vi "PMA Manuell Kalibrieren.vi"(8 "GT":bool, 10 "Kalibrieren":T4, 11 "AUTO STARTEN":bool) -> (2 "Wert im gültigen Bereich:":bool, 3 "Kalibrieren erfolgreich":bool)   [LabVIEW 2020, in "ABB-EL3000.lvlib" / "PMA.lvlib" / "Kalibrieren.lvlib"]
uses:
  Kalibrieren.lvlib
  Visualisierungs Elemente/Button.ctl
  Kalibrierung O2.ctl
  Visualisierungs Elemente/String - Ausgabefeld.ctl
  Visualisierungs Elemente/Zahlen-Ausgabefeld.ctl
  Analysator Definition/FGV Analysator Definition Aktionen.ctl
  Sprachverwaltung/FGV Aktion Tabelle zerlegen.ctl
  CalGas Aufschaltung/FGV CalGas Aktionen.ctl
  Linearisierung V2/Aktion Lin Daten aufarbeiten.ctl
  Allgemeine VI/FGV Uras26 Aktion.ctl
  Allgemeine VI/Allgemeine VI.lvlib
  Auto Kalibrieren/Auto Kalibrieren.lvlib
  Analysator Definition/Analysator Definition.lvlib
  CalGas Aufschaltung/CalGas Aufschaltung.lvlib
  Sprachverwaltung/Sprachverwaltung.lvlib
  Allgemein/allgemeine Sub-VIs.lvlib
  Linearisierung V2/Linearisierung v2.lvlib
panel:
  in  "Speichern":T1
  in  "Kalibrierwerte kopieren?:":bool
  out "Titelzeile":string
  out "Roh Wert O2:":T2 format="%.3f"
  out "Status":T3
  in  "Konzentration":sgl format="%#_5g"
  out "Messbereich":T3
  in  "STARTEN":bool
  in  "ABBRECHEN":T1
  # "Messbereich"
  # "%"
  # "Konzentration"
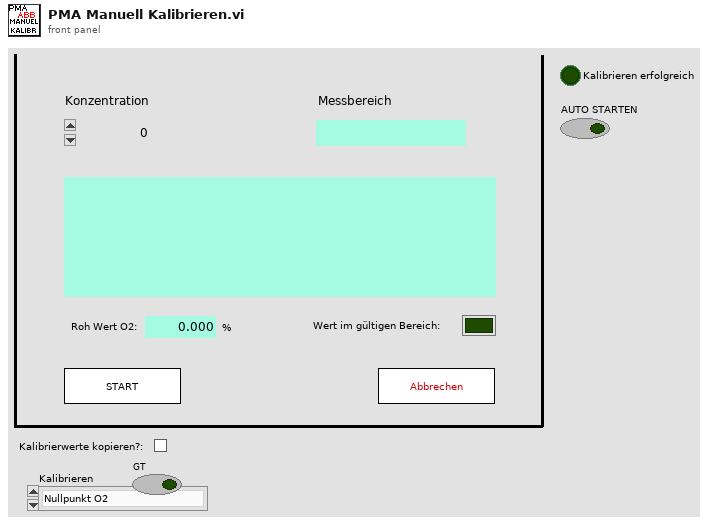
[diagram p1: front panel]
types:
  T1 = typedef "Button.ctl" = bool
  T2 = typedef "Zahlen-Ausgabefeld.ctl" = sgl
  T3 = typedef "String - Ausgabefeld.ctl" = string
  T4 = typedef "ABB-EL3000.lvlib/PMA.lvlib/Kalibrieren.lvlib/Kalibrierung O2.ctl" = enum16{"Nullpunkt O2", "Endpunkt O2"}
  T5 = typedef "Sprachverwaltung.lvlib/FGV Aktion Tabelle zerlegen.ctl" = enum16{"laden", "vereinzeln", "speichern"}
  T6 = enum8{"Enabled", "Disabled", "Disabled and Grayed Out"}
  T7 = typedef "Analysator Definition.lvlib/FGV Analysator Definition Aktionen.ctl" = enum16{"lesen", "MB setzen", "MB KAL setzen", "laden"}
  T8 = typedef "Linearisierung v2.lvlib/Aktion Lin Daten aufarbeiten.ctl" = enum16{"lesen", "Protkolldaten", "speichern", "laden", "EPA auswerten", "Tabelle schreiben", "Lin auswerten", "Tab init", "Stufentabelle", "EPA aktiviert", "Nachbehandlung laden", "Tabelle löschen", "Istwerte löschen", "Zeile löschen", "Zeile einfügen", "LIN aktiviert", "LIN/EPA aktiv laden", "EGAK Tab", "LIN übernehmen", "Tab init ohne Stufen"}
  T9 = typedef "CalGas Aufschaltung.lvlib/FGV CalGas Aktionen.ctl" = enum16{"lesen", "Analysator Auswahl", "Def.CalGas", "Aufschaltung CalGas", "laden", "speichern", "KAL extrahieren"}
  T10 = typedef "Linearisierung v2.lvlib/Lin-Polynom Daten.ctl" = cluster{"Messgerät":string, "Kalibrator (Gasteiler)":string, "Bearbeiter/in":string, "Komponente":string, "Zeitstempel":timestamp, "F_max gefordert (%)":sgl, "F_max in %":sgl, "F_max in ppm":sgl, "Vorschlag Ordnung":i32, "Polynom OK":bool, "Polynomkoeff.":dbl[], "Prüfgas Konzentration":dbl, "Pfad EPA":string, "Pfad_LIN":string, "Gasnummer:":u8, "Komponentenauswahl":T11, "Verdünnungsgas":T13, "Zeitdauer Stufe":T14, "Anzahl Stufen":T14, "F_max in % EPA":sgl, "F_max in ppm EPA":sgl, "F_max in % LIN":sgl, "F_max in ppm LIN":sgl, "Punkte umkehren":bool, "EPA Optionsfeld":T15, "Autolin Hovacal":T16, "Spanfactors":sgl[], "Kalibrierauswahl":T17, "Conditions:":T18, "Gasflaschen Nr.:":string, "Bottle Accuracy":dbl, "Konfig Gasflasche":T19, "Gasflasche":T20, "HovaCAL Flow AutoLin":T21, "MFC Output":T22, "Gas Ablaufdatum":timestamp, "Lin Modus":T23, "zusätzliche Zeitdauer Erster Punkt":sgl, "Offsets":sgl[]}
  T11 = typedef "Linearisierung v2.lvlib/KomponentenArray.ctl" = cluster{"Komponente:":T12, "Konzentration":dbl}[]
  T12 = typedef "Auswahlfeld.ctl" = u16
  T13 = typedef "Linearisierung v2.lvlib/Gasteiler.lvlib/Prüfgas in.ctl" = u16
  T14 = typedef "Zahlen-Eingabefeld.ctl" = sgl
  T15 = typedef "Linearisierung v2.lvlib/EPA Optionsfeld.ctl" = enum32{"Istwert", "Rohwert", "Linearisierter Wert"}
  T16 = typedef "Linearisierung v2.lvlib/Gasteiler.lvlib/HovaCal.lvlib/AutoLin Hovacal.ctl" = enum32{"Keine Auswahl", "Optionsauswahl 1", "Optionsauswahl 2"}
  T17 = typedef "Linearisierung v2.lvlib/Kalibrieroption.ctl" = u16
  T18 = typedef "Linearisierung v2.lvlib/Linearity verification 1065-307.lvlib/Condition.ctl" = u16
  T19 = typedef "System Einstellungen V2.lvlib/Konfig Gasflasche.ctl" = bool
  T20 = typedef "System Einstellungen V2.lvlib/Gasflasche Auswahl.ctl" = u16
  T21 = typedef "Linearisierung v2.lvlib/Gasteiler.lvlib/HovaCAL_Interface.lvlib/Controls.lvlib/Flow Einstellung.ctl" = cluster{"HovaCAL Flow Input Cluster":dbl}
  T22 = typedef "Linearisierung v2.lvlib/Gasteiler.lvlib/HovaCAL_Interface.lvlib/Controls.lvlib/Pump state.ctl" = cluster{"Run":bool}
  T23 = typedef "CalGas Aufschaltung.lvlib/Lin Modus.ctl" = u16
  T24 = typedef "CalGas Aufschaltung.lvlib/Definition CalGas Anzeige.ctl" = cluster{"Namen":T25, "Werte":T27, "Werte 2":T27, "Einheit":T28, "Messbereiche":T29}
  T25 = typedef "CalGas Aufschaltung.lvlib/CalGas-Namen.ctl" = cluster{"Name":T26, "Name 2":T26, "Name 3":T26, "Name 4":T26, "Name 5":T26, "Name 6":T26, "Name 7":T26, "Name 8":T26, "Name 9":T26, "Name 10":T26, "Name 11":T26, "Name 12":T26}
  T26 = typedef "String - Eingabefeld.ctl" = string
  T27 = typedef "CalGas Aufschaltung.lvlib/CalGas-Werte.ctl" = cluster{"Konzentration 1":T14, "Konzentration 2":T14, "Konzentration 3":T14, "Konzentration 4":T14, "Konzentration 5":T14, "Konzentration 6":T14, "Konzentration 7":T14, "Konzentration 8":T14, "Konzentration 9":T14, "Konzentration 10":T14, "Konzentration 11":T14, "Konzentration 12":T14}
  T28 = typedef "CalGas Aufschaltung.lvlib/CalGas-Einheit.ctl" = cluster{"Einheit 1":T12, "Einheit 2":T12, "Einheit 3":T12, "Einheit 4":T12, "Einheit 5":T12, "Einheit 6":T12, "Einheit 7":T12, "Einheit 8":T12, "Einheit 9":T12, "Einheit 10":T12, "Einheit 11":T12, "Einheit 12":T12}
  T29 = typedef "CalGas Aufschaltung.lvlib/CalGas-Messbereiche.ctl" = cluster{"Messbereich 1":T12, "Messbereich 2":T12, "Messbereich 3":T12, "Messbereich 4":T12, "Messbereich 5":T12, "Messbereich 6":T12, "Messbereich 7":T12, "Messbereich 8":T12, "Messbereich 9":T12, "Messbereich 10":T12, "Messbereich 11":T12, "Messbereich 12":T12}
  T30 = typedef "Analysator Definition.lvlib/Betriebsdaten Komponente.ctl" = cluster{"Namen":string[], "MB Namen":string[], "Einheit":string, "MB Aktuell":u16, "MB Endwert":u16, "CalGase":u16[], "MB für KAL":u16[], "CG für KAL":u16[]}
  T31 = typedef "ABB-EL3000.lvlib/Allgemeine VI.lvlib/FGV Uras26 Aktion.ctl" = enum16{"lesen", "CAL-Daten laden", "Messen", "Kalibrieren vorbereiten", "Kalibrieren", "CAL-Daten speichern", "Toleranz schreiben", "CAL-Daten kopieren"}
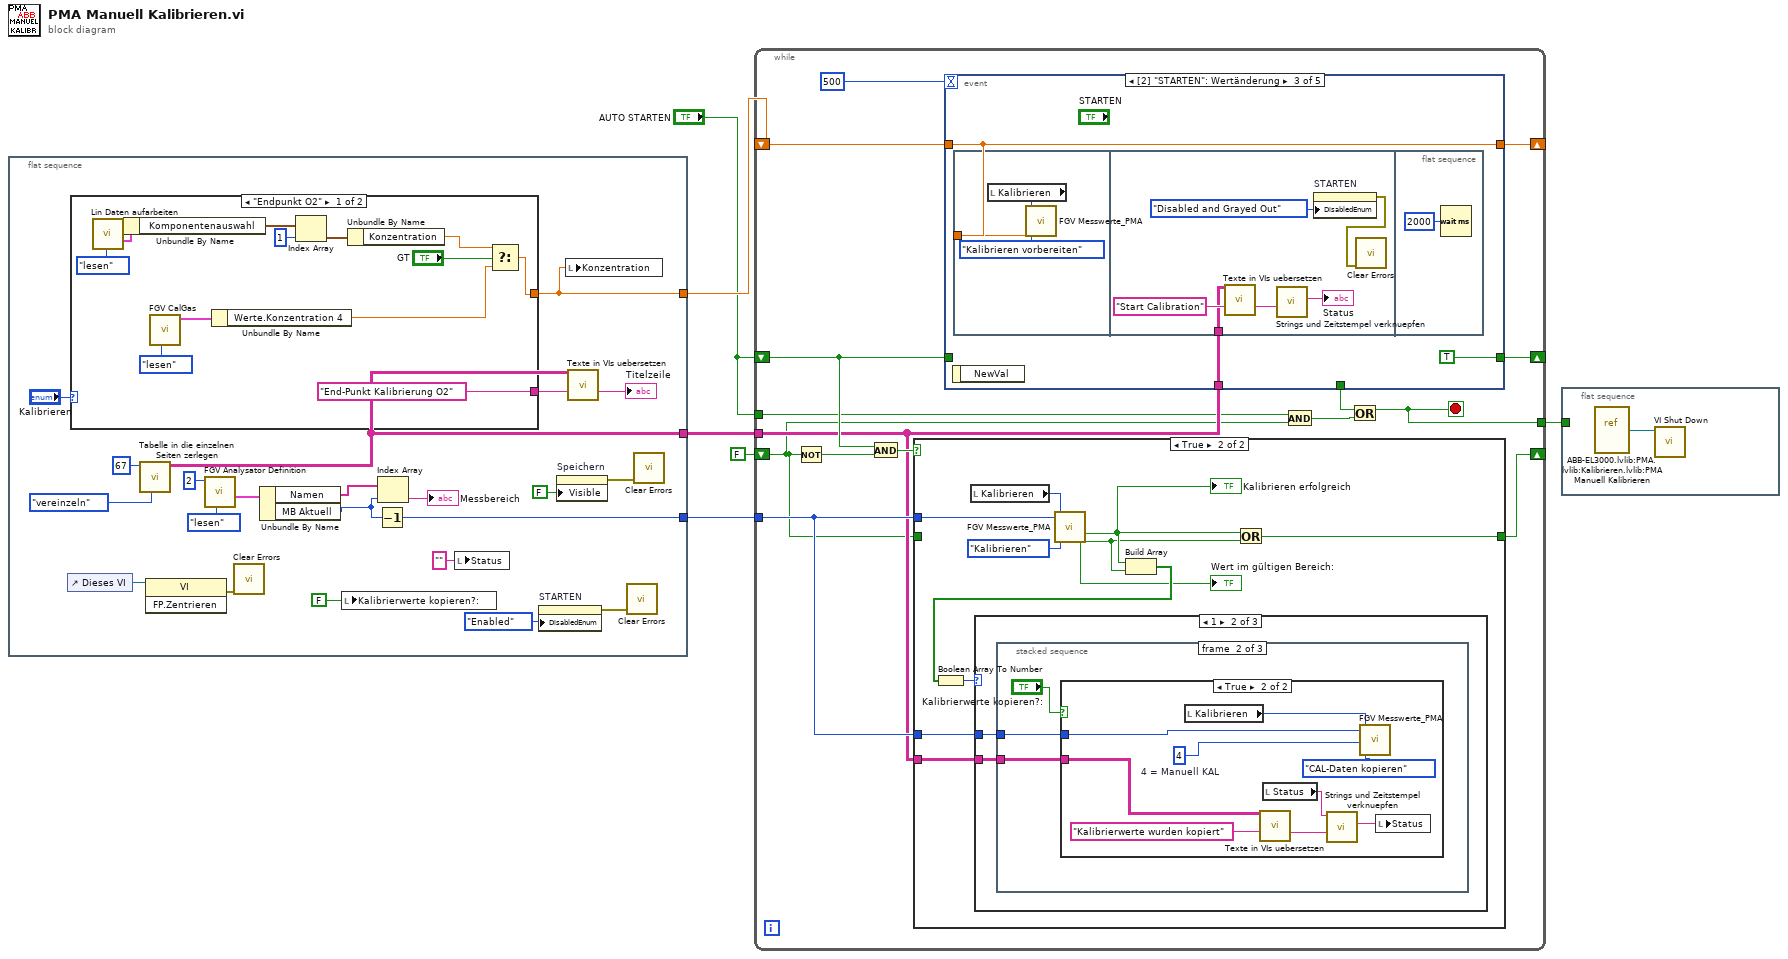
[diagram p0: block diagram]
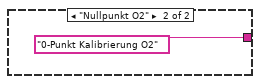
[diagram p2: hidden frame]
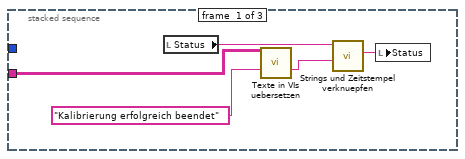
[diagram p5: hidden frame]
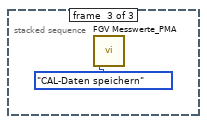
[diagram p7: hidden frame]
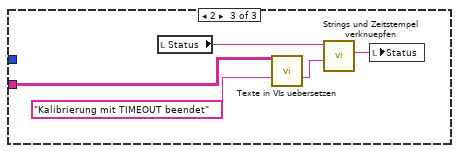
[diagram p8: hidden frame]
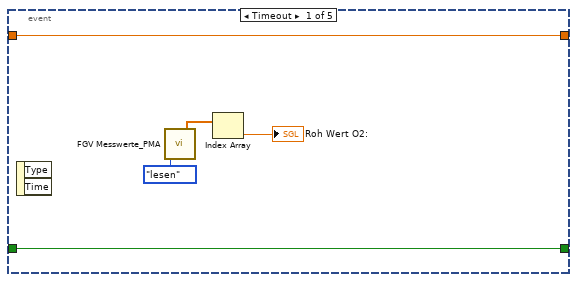
[diagram p9: hidden frame]
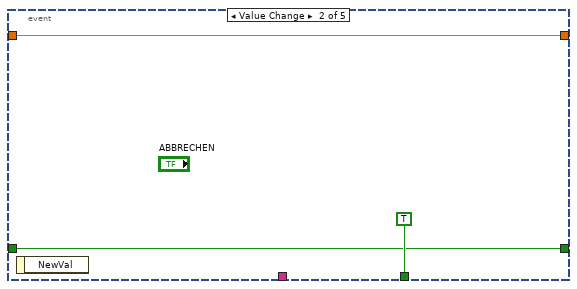
[diagram p10: hidden frame]
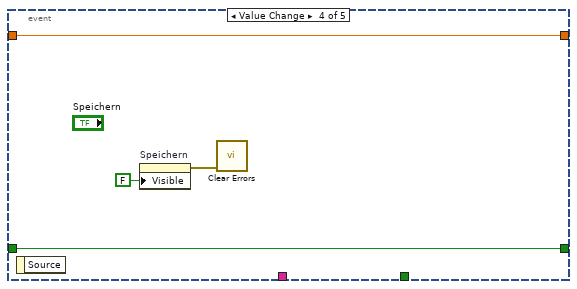
[diagram p11: hidden frame]
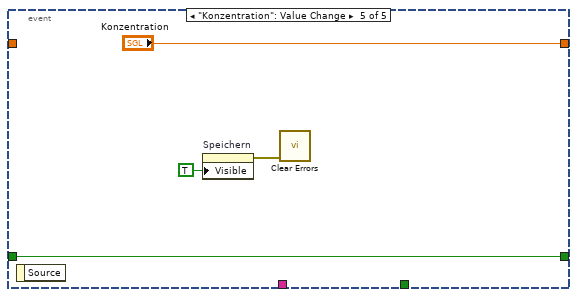
[diagram p12: hidden frame]
diagram:
  n1 = flat-sequence {
    tunnel: [w15] -> w5
    tunnel: [w8] -> w4
    tunnel: [w9] -> w3
    frame #0 {
      n2 = control-ref of="Dieses VI"() -> (w14:refnum<vi>)
      n3 = case shown="\"Endpunkt O2\"" "Kalibrieren" {
        tunnel: ["End-Punkt Kalibrierung O2" "0-Punkt Kalibrierung O2"] -> w11
        tunnel: [w29 _] -> w8
        frame "Endpunkt O2" {
          n4 = call "Lin Daten aufarbeiten.vi"("Aktionen"=Aktion_Lin_Daten_aufarbeiten."lesen") -> ("Lin-Polynom"=w32:T10)  [unwired: 16 in, 10 out]
          n5 = Unbundle By Name(w32) -> ("Komponentenauswahl"=w33:T11)
          n6 = call "FGV CalGas.vi"("Aktionen"=FGV_CalGas_Aktionen."lesen") -> ("Def.CalGas"=w38:T24)  [unwired: 6 in, 4 out]
          n7 = Unbundle By Name(w38) -> ("Werte.Konzentration 4"=w30:T14)
          n8 = Index Array(array=w33, index=1 ("Index")) -> (element=w35:cluster{"Komponente:":T12, "Konzentration":dbl})
          n9 = Unbundle By Name(w35) -> ("Konzentration"=w36:dbl)
          n10 = Select(t=w36, s="GT", f=w30) -> (s? t:f=w29:dbl)
        }
        frame "Nullpunkt O2" {
        }
      }
      n11 = call "Tabelle in die einzelnen Seiten zerlegen.vi"("Aktion"=FGV_Aktion_Tabelle_zerlegen."vereinzeln", "Index (Seite)"=67) -> ("Sprachliste"=w9:string[][])  [unwired: 7 in, 2 out]
      n12 = invoke class="VI" method="FP.Zentrieren"(reference=w14) -> (error out=w13:errorcluster)  [unwired: 2 in, 2 out]
      n13 = call "FGV Analysator Definition.vi"("Aktionen"=FGV_Analysator_Definition_Aktionen."lesen", "Komponente"=2) -> ("Betriebsdaten Komponente"=w24:T30)  [unwired: 5 in, 4 out]
      n14 = call <vilib>:"Clear Errors.vi"("error in (no error)"=w13) -> ()  [unwired: 5 in, 2 out]
      n15 = Unbundle By Name(w24) -> ("Namen"=w25:string[], "MB Aktuell"=w20:u16)
      n16 = local write "Kalibrierwerte kopieren?:"(FALSE) -> ()
      n17 = Decrement(x=w20) -> (x-1=w15:u16)
      n18 = Index Array(array=w25, index=w20) -> (element=→"Messbereich":string)
      n19 = local write "Status"(T3 "" ("Status")) -> ()
      n20 = property on="STARTEN" class="Bool."("DisabledEnum"=T6."Enabled" ("Deaktiviert")) -> (error out=w16:errorcluster)  [unwired: 2 in, 1 out]
      n21 = property on="Speichern" class="Bool."("Visible"=FALSE ("Sichtbar")) -> (error out=w19:errorcluster)  [unwired: 2 in, 1 out]
      n22 = local write "Konzentration"(w8) -> ()
      n23 = call "Texte in VIs uebersetzen.vi"("Sprachliste"=w9, "String zum Übersetzen"=w11) -> ("String zum Übersetzen"=→"Titelzeile":string)  [unwired: 9 in, 4 out]
      n24 = call <vilib>:"Clear Errors.vi"("error in (no error)"=w16) -> ()  [unwired: 5 in, 2 out]
      n25 = call <vilib>:"Clear Errors.vi"("error in (no error)"=w19) -> ()  [unwired: 5 in, 2 out]
    }
  }
  n26 = while {
    shift-right: [w55] -> _
    shift-left: "AUTO STARTEN" -> [w53]
    tunnel: w5 -> [w50]
    shift-right: [w43] -> _
    shift-left: FALSE -> [w42]
    tunnel: [w46] -> w6
    shift-right: [w49] -> _
    shift-left: w4 -> [w48]
    tunnel: w3 -> [w47]
    tunnel: "AUTO STARTEN" -> [w44]
    stop <- w46 stop-if-true
    n27 = Not(x=w42) -> (.not. x?=w54:bool)
    n28 = And(x=w53, y=w54) -> (x .and. y?=w52:bool)
    n29 = case shown="True" w52 {
      tunnel: w50 -> [_ w61]
      tunnel: [w57 w67] -> w43
      tunnel: w42 -> [w57 _]
      tunnel: w50 -> [_ w60]
      tunnel: w47 -> [_ w58]
      frame False {
      }
      frame True {
        n30 = local read "Kalibrieren"() -> (w62:T4)
        n31 = call "FGV Messwerte_PMA.vi"("Messbereich"=w61, "Kalibrieren"=w62, "Aktion"=FGV_Uras26_Aktion."Kalibrieren") -> ("im gültigen Bereich"=→"Wert im gültigen Bereich:":bool, "Kalibrieren erfolgreich"=w66:bool, "CAL TimeOut"=w65:bool)  [unwired: 17 in, 5 out]
        "Kalibrieren erfolgreich" <- w66
        n32 = Build Array(w66, w65) -> (w64:bool[])
        n33 = Boolean Array To Number(Boolean array=w64) -> (number=w63:u32)
        n34 = case shown="1" w63 {
          tunnel: w60 -> [_ w70 _]
          tunnel: w58 -> [_ w69 w89]
          frame 0, Default {
          }
          frame 1 {
            n35 = stacked-sequence {
              tunnel: w70 -> [_ w77 _]
              tunnel: w69 -> [w71 w76 _]
              frame #0 {
                n36 = local read "Status"() -> (w74:T3)
                n37 = call "Texte in VIs uebersetzen.vi"("Sprachliste"=w71, "String zum Übersetzen"="Kalibrierung erfolgreich beendet" ("String 1 hinzufügen")) -> ("String zum Übersetzen"=w72:string)  [unwired: 9 in, 4 out]
                n38 = call "Strings und Zeitstempel verknuepfen.vi"("String 1 hinzufügen"=w72, "Eingagns String"=w74) -> ("Verknüpfter String"=w75:string)  [unwired: 9 in]
                n39 = local write "Status"(w75) -> ()
              }
              frame #1 {
                n40 = case shown="True" "Kalibrierwerte kopieren?:" {
                  tunnel: w77 -> [_ w83]
                  tunnel: w76 -> [_ w79]
                  frame False {
                  }
                  frame True {
                    w82 = u16 4  # 4 = Manuell KAL
                    n41 = local read "Kalibrieren"() -> (w84:T4)
                    n42 = call "Texte in VIs uebersetzen.vi"("Sprachliste"=w79, "String zum Übersetzen"="Kalibrierwerte wurden kopiert" ("String 1 hinzufügen")) -> ("String zum Übersetzen"=w80:string)  [unwired: 9 in, 4 out]
                    n43 = local read "Status"() -> (w86:T3)
                    n44 = call "Strings und Zeitstempel verknuepfen.vi"("String 1 hinzufügen"=w80, "Eingagns String"=w86) -> ("Verknüpfter String"=w87:string)  [unwired: 9 in]
                    n45 = call "FGV Messwerte_PMA.vi"("Messbereich"=w83, "Zielmessbereich"=w82, "Kalibrieren"=w84, "Aktion"=FGV_Uras26_Aktion."CAL-Daten kopieren") -> ()  [unwired: 16 in, 8 out]
                    n46 = local write "Status"(w87) -> ()
                  }
                }
              }
              frame #2 {
                n47 = call "FGV Messwerte_PMA.vi"("Aktion"=FGV_Uras26_Aktion."CAL-Daten speichern") -> ()  [unwired: 19 in, 8 out]
              }
            }
          }
          frame 2 {
            n48 = local read "Status"() -> (w93:T3)
            n49 = call "Texte in VIs uebersetzen.vi"("Sprachliste"=w89, "String zum Übersetzen"="Kalibrierung mit TIMEOUT beendet" ("String 1 hinzufügen")) -> ("String zum Übersetzen"=w90:string)  [unwired: 9 in, 4 out]
            n50 = call "Strings und Zeitstempel verknuepfen.vi"("String 1 hinzufügen"=w90, "Eingagns String"=w93) -> ("Verknüpfter String"=w92:string)  [unwired: 9 in]
            n51 = local write "Status"(w92) -> ()
          }
        }
        n52 = Or(x=w66, y=w65) -> (x .or. y?=w67:bool)
      }
    }
    n53 = event shown="[2] \"STARTEN\": Wertänderung" {
      selector: _ -> [_ _ _ _ _]
      dyn-events: _ -> [_ _ _ _ _]
      timeout: 500 -> [_ _ _ _ _]
      tunnel: [_ TRUE ("ABBRECHEN") _ _ _] -> w51
      tunnel: [w98 w100 TRUE ("STARTEN") w117 w119] -> w55
      tunnel: w53 -> [w98 w100 _ w117 w119]
      tunnel: [w95 w99 w103 w118 "Konzentration"] -> w49
      tunnel: w48 -> [w95 w99 w103 w118 _]
      tunnel: w47 -> [_ _ w102 _ _]
      event Timeout {
        n54 = event-data() -> ()  [unwired: 1 in, 2 out]
        n55 = call "FGV Messwerte_PMA.vi"("Aktion"=FGV_Uras26_Aktion."lesen") -> ("Rohwerte"=w96:sgl[])  [unwired: 19 in, 7 out]
        n56 = Index Array(array=w96) -> (element=→"Roh Wert O2:":sgl)  [unwired: 1 in]
      }
      event Value Change {
        n57 = event-data() -> ()  [unwired: 1 in, 1 out]
      }
      event "STARTEN": Value Change {
        n58 = event-data() -> ()  [unwired: 1 in, 1 out]
        n59 = flat-sequence {
          tunnel: w103 -> [w105]
          tunnel: w102 -> [w108]
          frame #0 {
            n60 = local read "Kalibrieren"() -> (w106:T4)
            n61 = call "FGV Messwerte_PMA.vi"("Prüfgaskonz."=w105, "Kalibrieren"=w106, "Aktion"=FGV_Uras26_Aktion."Kalibrieren vorbereiten") -> ()  [unwired: 17 in, 8 out]
          }
          frame #1 {
            n62 = call "Texte in VIs uebersetzen.vi"("Sprachliste"=w108, "String zum Übersetzen"="Start Calibration" ("String 1 hinzufügen")) -> ("String zum Übersetzen"=w109:string)  [unwired: 9 in, 4 out]
            n63 = call "Strings und Zeitstempel verknuepfen.vi"("String 1 hinzufügen"=w109) -> ("Verknüpfter String"=→"Status":string)  [unwired: 10 in]
            n64 = property on="STARTEN" class="Bool."("DisabledEnum"=T6."Disabled and Grayed Out" ("Deaktiviert")) -> (error out=w111:errorcluster)  [unwired: 2 in, 1 out]
            n65 = call <vilib>:"Clear Errors.vi"("error in (no error)"=w111) -> ()  [unwired: 5 in, 2 out]
          }
          frame #2 {
            n66 = Wait (ms)(milliseconds to wait=u32 2000 ("Zu wartende ms")) -> ()  [unwired: 1 out]
          }
        }
      }
      event Value Change {
        n67 = event-data() -> ()  [unwired: 1 in, 1 out]
        n68 = property on="Speichern" class="Bool."("Visible"=FALSE ("Sichtbar")) -> (error out=w115:errorcluster)  [unwired: 2 in, 1 out]
        n69 = call <vilib>:"Clear Errors.vi"("error in (no error)"=w115) -> ()  [unwired: 5 in, 2 out]
      }
      event "Konzentration": Value Change {
        n70 = event-data() -> ()  [unwired: 1 in, 1 out]
        n71 = property on="Speichern" class="Bool."("Visible"=TRUE ("Sichtbar")) -> (error out=w120:errorcluster)  [unwired: 2 in, 1 out]
        n72 = call <vilib>:"Clear Errors.vi"("error in (no error)"=w120) -> ()  [unwired: 5 in, 2 out]
      }
    }
    n73 = And(x=w44, y=w42) -> (x .and. y?=w45:bool)
    n74 = Or(x=w51, y=w45) -> (x .or. y?=w46:bool)
  }
  n75 = flat-sequence {
    tunnel: w6 -> [_]
    frame #0 {
      n76 = vi-ref "ABB-EL3000.lvlib:PMA.lvlib:Kalibrieren.lvlib:PMA Manuell Kalibrieren.vi"() -> (w123:refnum<vi>)
      n77 = call "VI Shut Down.vi"("VI Referenz"=w123) -> ()  [unwired: 11 in]
    }
  }
